vi "Generate DGML Reference string.vi"(8 "error in (no error)":errorcluster, 10 "Name":string, 11 "String in":string) -> (0 "error out":errorcluster, 3 "String out":string)   [LabVIEW 2018, in "DGML creation.lvlib"]
uses:
  DGML creation.lvlib
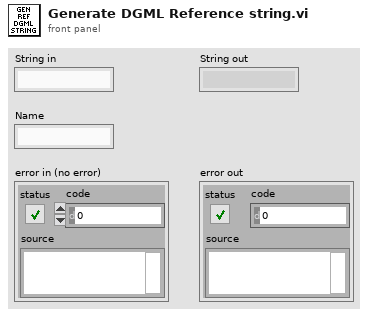
[diagram p1: front panel]
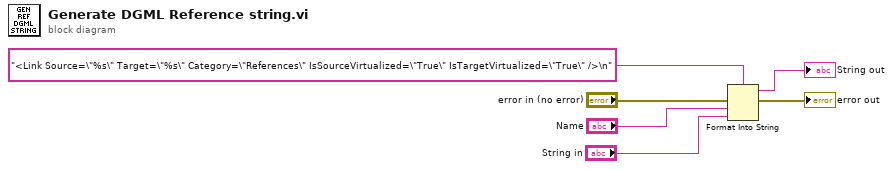
[diagram p0: block diagram]
diagram:
  n1 = Format Into String(format string="<Link Source=\"%s\" Target=\"%s\" Category=\"References\" IsSourceVirtualized=\"True\" IsTargetVirtualized=\"True\" />\n", error in="error in (no error)", "Name", "String in") -> (resulting string=→"String out":string, error out=→"error out":errorcluster)  [unwired: 1 in]
